vi "VI Reference To IWin32Window Reference.vi"(8 "error in (no error)":errorcluster, 11 "VI Reference":refnum<vi>) -> (0 "error out":errorcluster, 3 "System.Windows.Forms.IWin32Window":refnum<k24>)   [LabVIEW 2021]
doc: "This VI obtains a IWin32Window Reference for the VI Front Panel that is specified by the VI Reference.\n\n<b>REFERENCE</b> : https://forums.ni.com/t5/LabVIEW/Make-NET-called-Print-Dialog-frontmost/td-p/219217"
uses:
  System.Windows.Forms
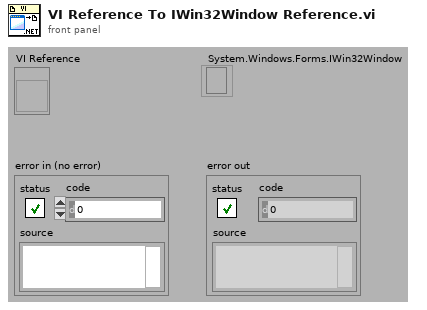
[diagram p1: front panel]
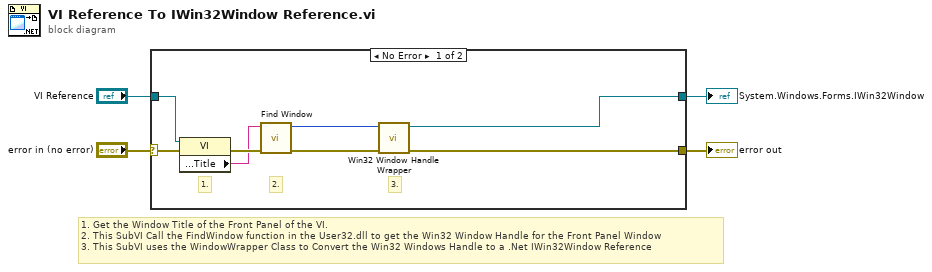
[diagram p0: block diagram]
diagram:
  # "1. Get the Window Title of the Front Panel of the VI.\n2. This SubVI Call the FindWindow function in the User32.dll to get the Win32 Window Handle for the Front Panel Window\n3. This SubVI uses the WindowWrapper Class to Convert the Win32 Windows Handle to a .Net IWin32Window Reference"
  n1 = case shown="No Error" "error in (no error)" {
    selector: "error in (no error)" -> [w5 w13]
    tunnel: [w12 _] -> w4
    tunnel: "VI Reference" -> [w7 _]
    tunnel: [w6 w13] -> w2
    frame No Error {
      # "3."
      # "2."
      # "1."
      n2 = property class="VI"(reference=w7, error in=w5) -> (error out=w9:errorcluster, "Front Panel.Title"=w8:string)  [unwired: 1 out]
      n3 = call "Find Window.vi"("error in (no error)"=w9, "Window Name"=w8) -> ("error out"=w11:errorcluster, "Win32 Window Handle"=w10:i32)  [unwired: 8 in]
      n4 = call "Win32 Window Handle Wrapper.vi"("error in (no error)"=w11, "Win32 Window Handle"=w10) -> ("error out"=w6:errorcluster, "System.Windows.Forms.IWin32Window"=w12:refnum<k24>)  [unwired: 8 in]
    }
    frame Error {
    }
  }
  "System.Windows.Forms.IWin32Window" <- w4
  "error out" <- w2
